vi "Nonlinear System Prep.vi"(4 "list of variables":i32[](array[numeric])=[0, 0], 5 "table":i32[][][](array[numeric]), 6 "accuracy":dbl format="%.2f", 7 "Start":dbl[](array[numeric]) format="%.2f", 8 "h":dbl format="%.2f", 9 "Diagonal h":dbl[][](array[numeric]) format="%.2f", 10 "result":dbl[][](array[numeric]) format="%.2f", 11 "length of Start":i32) -> (0 "error":bool, 1 "F(X)":dbl[](array[numeric]) format="%.2f", 3 "Start new":dbl[](array[numeric]) format="%.2f")   [LabVIEW 2020, in "NI_Gmath.lvlib"]
uses:
  NI_Gmath.lvlib
  NI_AALBase.lvlib
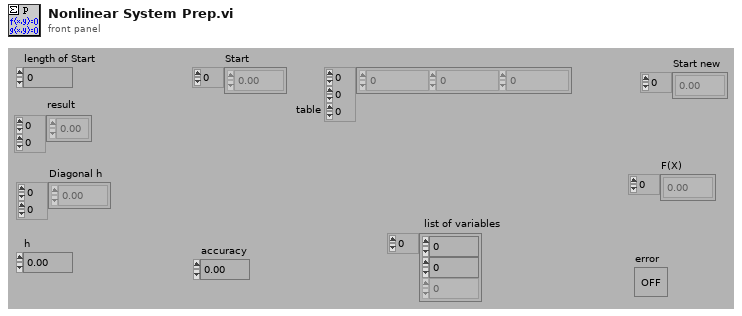
[diagram p1: front panel]
types:
  T1 = typedef "NI_Matrix.lvlib/RealMatrix.ctl" = dbl[][]
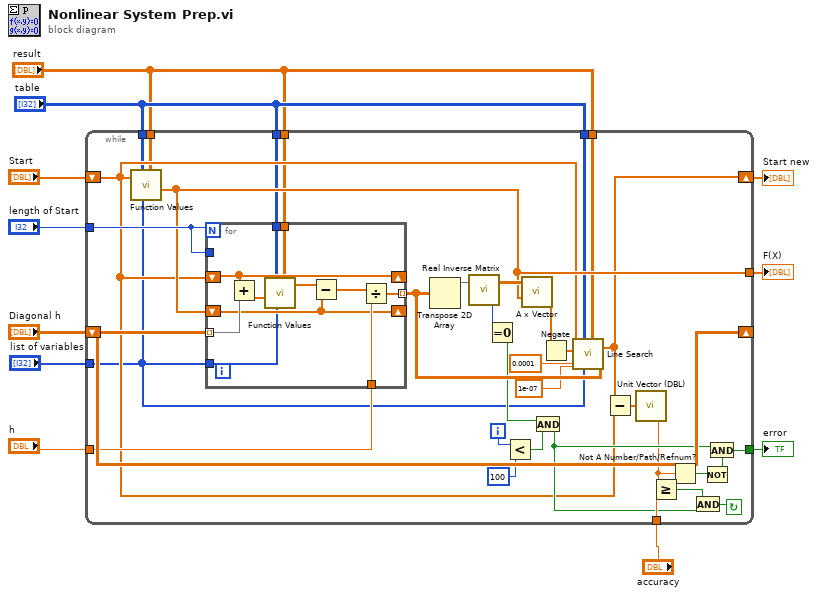
[diagram p0: block diagram]
diagram:
  n1 = while {
    tunnel: [w27] -> w10
    tunnel: [w22] -> w5
    tunnel: "accuracy" -> [w42]
    tunnel: "h" -> [w43]
    tunnel: "length of Start" -> [w44]
    shift-left: "Diagonal h" -> [w45]
    shift-right: [w45] -> _
    shift-left: "Start" -> [w20]
    shift-right: [w21] -> w11
    tunnel: "table" -> [w18]
    tunnel: "result" -> [w17]
    tunnel: "list of variables" -> [w14]
    tunnel: "table" -> [w16]
    tunnel: "result" -> [w15]
    tunnel: "table" -> [w13]
    tunnel: "result" -> [w12]
    i -> [w29]
    stop <- w33 continue-if-true
    n2 = call "Function Values.vi"("result"=w17, "list of variables"=w14, "table"=w18, "X"=w20) -> ("F(X)"=w22:dbl[])  [unwired: 7 in]
    n3 = for {
      N: w44 -> [_]
      tunnel: w44 -> [_]
      shift-right: [w54] -> _
      shift-left: w20 -> [w54]
      tunnel: w45 -> [w56] mode=indexing
      shift-right: [w50] -> _
      shift-left: w22 -> [w50]
      tunnel: w43 -> [w52]
      tunnel: [w49] -> w41 mode=indexing
      tunnel: w16 -> [w48]
      tunnel: w15 -> [w47]
      tunnel: w14 -> [w46]
      n4 = Add(x=w54, y=w56) -> (x+y=w55:dbl[])
      n5 = call "Function Values.vi"("result"=w47, "list of variables"=w46, "table"=w48, "X"=w55) -> ("F(X)"=w53:dbl[])  [unwired: 7 in]
      n6 = Subtract(x=w53, y=w50) -> (x-y=w51:dbl[])
      n7 = Divide(x=w51, y=w52) -> (x/y=w49:dbl[])
    }
    n8 = Transpose 2D Array(2D array=w41) -> (transposed array=w35:dbl[][])
    n9 = call "Real Inverse Matrix.vi"("Input Matrix"=w35) -> ("error"=w32:i32, "Inverse Matrix"=w40:T1)  [unwired: 1 in]
    n10 = Equal To 0?(x=w32) -> (x = 0?=w31:bool)
    n11 = Less?(x=w29, y=100) -> (x < y?=w30:bool)
    n12 = call "A x Vector.vi"("Vector"=w22, "A"=w40) -> ("A x Vector"=w39:dbl[])  [unwired: 1 out]
    n13 = And(x=w31, y=w30) -> (x .and. y?=w28:bool)
    n14 = Negate(x=w39) -> (-x=w38:dbl[])
    n15 = call "Line Search.vi"("J"=w41, "result"=w12, "list of variables"=w14, "table"=w13, "TOLX"=1e-07, "alpha"=0.0001, "P"=w38, "X"=w20) -> ("X (new)"=w21:dbl[])  [unwired: 2 in, 1 out]
    n16 = Subtract(x=w21, y=w20) -> (x-y=w19:dbl[])
    n17 = call "Unit Vector (DBL).vi"("Input Vector"=w19) -> ("norm"=w25:dbl)  [unwired: 8 in, 2 out]
    n18 = Greater Or Equal?(x=w25, y=w42) -> (x >= y?=w26:bool)
    n19 = Not A Number/Path/Refnum?(number/path/refnum=w25) -> (NaN/Path/Refnum?=w24:bool)
    n20 = And(x=w26, y=w28) -> (x .and. y?=w33:bool)
    n21 = Not(x=w24) -> (.not. x?=w23:bool)
    n22 = And(x=w28, y=w23) -> (x .and. y?=w27:bool)
  }
  "Start new" <- w11
  "error" <- w10
  "F(X)" <- w5
